vi "initializeBK.vi"(11 "VISA resource name":refnum<visa-resource-name>="COM1") -> (0 "error out":errorcluster, 2 "Device ID":string, 3 "VISA resource name out":refnum<visa-resource-name>)   [LabVIEW 2021]
panel:
  out "return count":u32
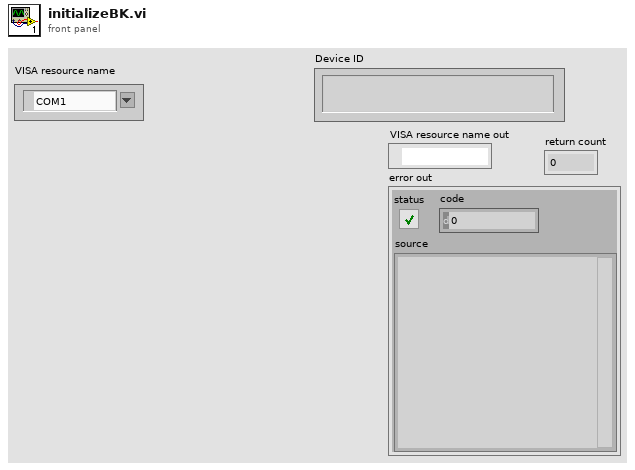
[diagram p1: front panel]
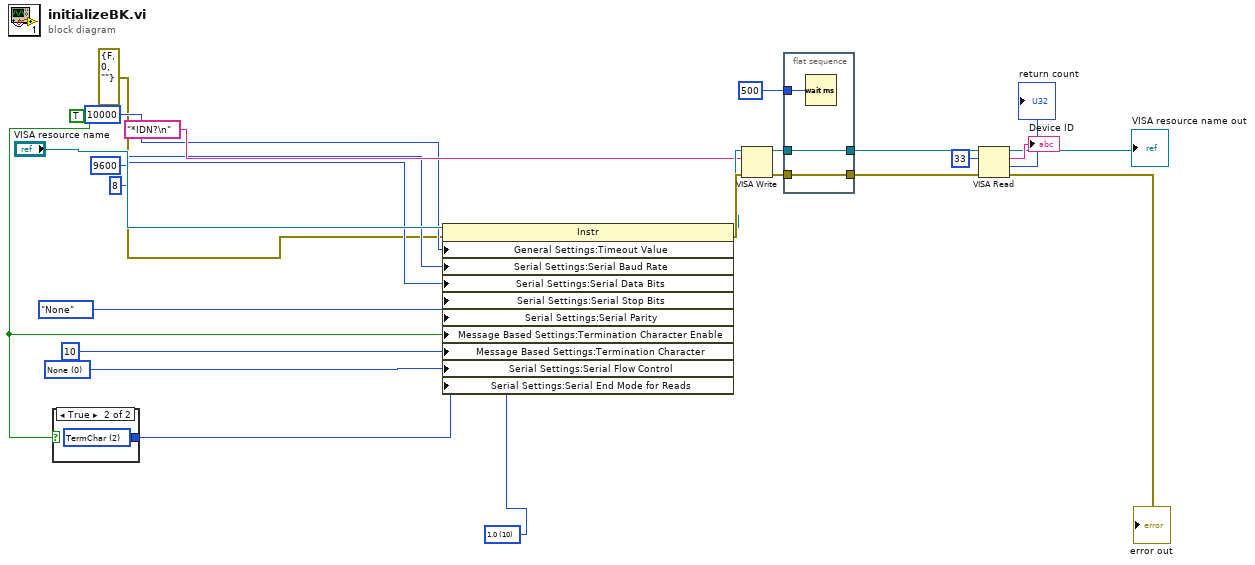
[diagram p0: block diagram]
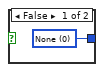
[diagram p2: hidden frame]
diagram:
  w2 = u16 0 items=["None", "XON/XOFF", "RTS/CTS", "XON/XOFF & RTS/CTS", "DTR/DSR", "XON/XOFF & DTR/DSR"] ("flow control (0:none)")
  w3 = u16 10 items=["1.0"=10, "1.5"=15, "2.0"=20] ("stop bits (10: 1 bit)")
  w8 = TRUE ("Enable Termination\nChar (T)")
  n1 = case shown="True" w8 {
    tunnel: [w25 w26] -> w1
    frame False {
      w25 = u16 0 items=["None", "LastBit", "TermChar"] ("Serial Settings:Serial End Mode for Reads")
    }
    frame True {
      w26 = u16 2 items=["None", "LastBit", "TermChar"] ("Serial Settings:Serial End Mode for Reads")
    }
  }
  n2 = property class="Instr"(reference="VISA resource name", error in=errorcluster {"status"=FALSE, "code"=0, "source"=""} ("error in (no error)"), "General Settings:Timeout Value"=u32 10000 ("timeout (10sec)"), "Serial Settings:Serial Baud Rate"=u32 9600 ("baud rate (9600)"), "Serial Settings:Serial Data Bits"=u16 8 ("data bits (8)"), "Serial Settings:Serial Stop Bits"=w3, "Serial Settings:Serial Parity"=enum16{"None", "Odd", "Even", "Mark", "Space"}."None" ("parity (0:none)"), "Message Based Settings:Termination Character Enable"=w8, "Message Based Settings:Termination Character"=u8 10 ("termination char\n(0xA = '\\n' = LF)"), "Serial Settings:Serial Flow Control"=w2, "Serial Settings:Serial End Mode for Reads"=w1) -> (reference out=w22:refnum<visa-resource-name>, error out=w23:errorcluster)
  n3 = VISA Write(VISA resource name=w22, write buffer="*IDN?\n" ("Command"), error in (no error)=w23) -> (VISA resource name out=w20:refnum<visa-resource-name>, error out=w21:errorcluster)  [unwired: 1 out]
  n4 = flat-sequence {
    tunnel: w21 -> [w28]
    tunnel: [w28] -> w13
    tunnel: w20 -> [w27]
    tunnel: [w27] -> w14
    tunnel: u32 500 ("delay before read (ms)") -> [w29]
    frame #0 {
      n5 = Wait (ms)(milliseconds to wait=w29) -> ()  [unwired: 1 out]
    }
  }
  n6 = VISA Read(VISA resource name=w14, byte count=u32 33, error in (no error)=w13) -> (VISA resource name out=→"VISA resource name out":refnum<visa-resource-name>, read buffer=→"Device ID":string, return count=→"return count":u32, error out=→"error out":errorcluster)
